vi "Swap (No Check).vi"(8 "error in (no error)":errorcluster, 10 "Pointer b":refnum<class "Pointer.lvclass">, 11 "Pointer a":refnum<class "Pointer.lvclass">) -> (0 "error out":errorcluster, 2 "Pointer b":refnum<class "Pointer.lvclass">, 3 "Pointer a":refnum<class "Pointer.lvclass">)   [LabVIEW 2017, in "Memory Manager.lvlib" / "Pointer.lvclass"]
doc: "Swaps the address of the two provided <b>pointers</b>. This cannot be used with external pointers created via the Encapsulate method.\n\n<b>Note:</b> This VI is <b>unsafe</b>.\n\nUnsafe means that this function does not evaluate the size parameter of <b>pointer a</b> and <b>pointer b</b> before peforming a memory read/write. Reading/writing more data to a pointer than it has allocated can corrupt or crash LabVIEW."
uses:
  Pointer.lvclass
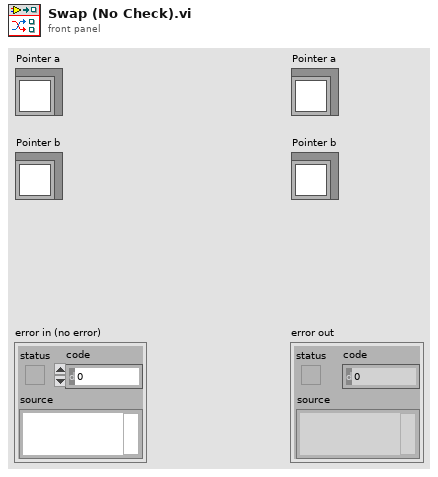
[diagram p1: front panel]
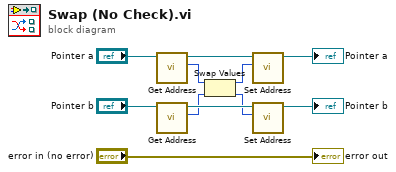
[diagram p0: block diagram]
diagram:
  n1 = call "Get Address.vi"("Pointer in"="Pointer a") -> ("address"=w9:u64, "Pointer out"=w7:refnum<class "Pointer.lvclass">)  [unwired: 9 in]
  n2 = call "Get Address.vi"("Pointer in"="Pointer b") -> ("address"=w6:u64, "Pointer out"=w8:refnum<class "Pointer.lvclass">)  [unwired: 9 in]
  n3 = Swap Values(12:w9, 14:w6) -> (1:w4:u64, 3:w5:u64)  [unwired: 1 in]
  n4 = call "Set Address.vi"("address"=w4, "Pointer in"=w7) -> ("Pointer out"=→"Pointer a":refnum<class "Pointer.lvclass">)  [unwired: 9 in]
  n5 = call "Set Address.vi"("address"=w5, "Pointer in"=w8) -> ("Pointer out"=→"Pointer b":refnum<class "Pointer.lvclass">)  [unwired: 9 in]
  "error out" <- "error in (no error)"
